vi "Tektronix Model Check.vi"(8 "error in (no error)":errorcluster, 9 "Command String":string, 10 "Oscilloscope Model Tests (3: RF Model?)":u16(ring)=3 items=["Two-channel?", "Digital Model?", "Four-channel?", "RF Model?"], 11 "VISA resource name":refnum<visa-resource-name>) -> (0 "error out":errorcluster, 3 "VISA resource name out":refnum<visa-resource-name>)   [LabVIEW 2017, in "Tektronix DPO MSO 2000 4000 Series.lvlib"]
doc: "Performs a model check on the instrument to verify it supports the commandset that is being written to it. The VI also writes the input command to the instrument."
uses:
  Tektronix DPO MSO 2000 4000 Series.lvlib
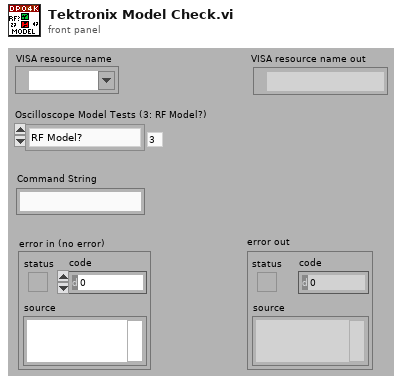
[diagram p1: front panel]
types:
  T1 = typedef "Tektronix DPO MSO 2000 4000 Series.lvlib/Extended User Data.ctl" = cluster{"DPO MSO Series Model":u16}
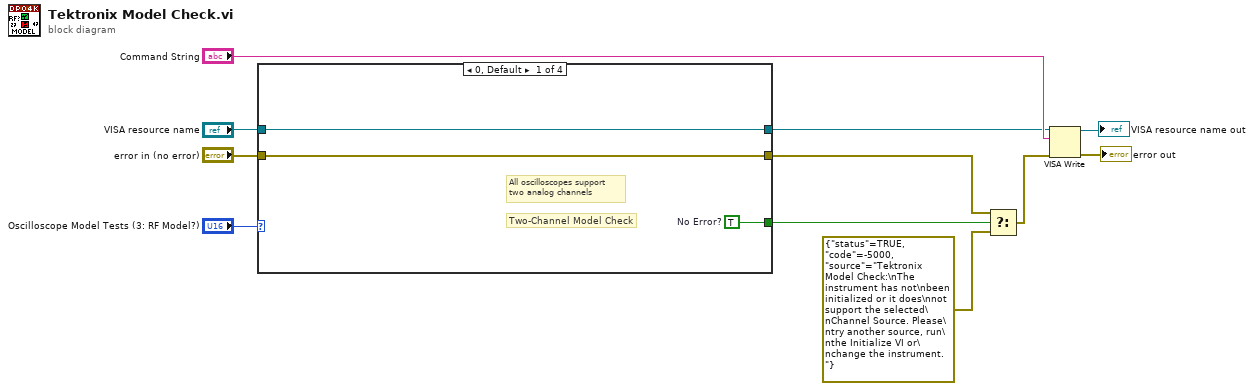
[diagram p0: block diagram]
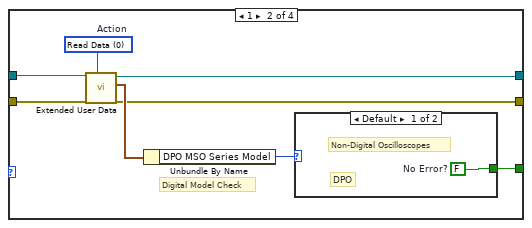
[diagram p2: hidden frame]
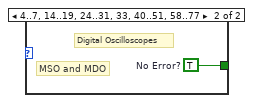
[diagram p3: hidden frame]
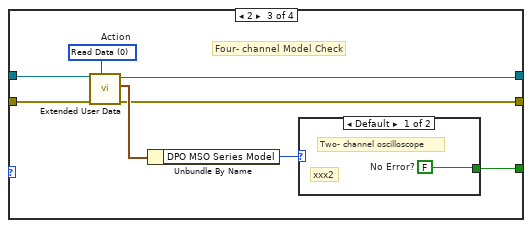
[diagram p4: hidden frame]
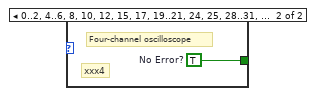
[diagram p5: hidden frame]
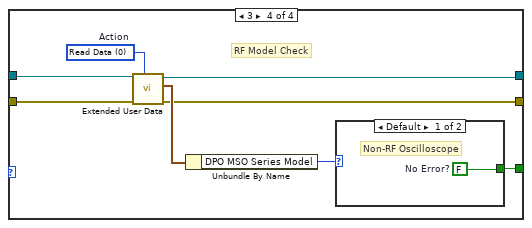
[diagram p6: hidden frame]
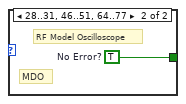
[diagram p7: hidden frame]
diagram:
  n1 = case shown="0, Default" "Oscilloscope Model Tests (3: RF Model?)" {
    tunnel: "VISA resource name" -> [w14 w19 w29 w39]
    tunnel: "error in (no error)" -> [w13 w18 w28 w38]
    tunnel: [w14 w17 w27 w37] -> w7
    tunnel: [w13 w16 w26 w35] -> w6
    tunnel: [w12 w22 w32 w42] -> w5
    frame 0, Default {
      w12 = TRUE  # No Error?
      # "All oscilloscopes support\ntwo analog channels"
      # "Two-Channel Model Check"
    }
    frame 1 {
      w21 = 0 items=["Read Data", "Write Data", "Clear Data", "Clear ALL Data"]  # Action
      # "Digital Model Check"
      n2 = call "Extended User Data.vi"("Action (1: Write Data)"=w21, "error in (no error)"=w18, "VISA resource name"=w19) -> ("error out"=w16:errorcluster, "User Data Out"=w20:T1, "VISA resource name out"=w17:refnum<visa-resource-name>)  [unwired: 6 in]
      n3 = Unbundle By Name(w20) -> ("DPO MSO Series Model"=w15:u16)
      n4 = case shown="Default" w15 {
        tunnel: [w23 w24] -> w22
        frame Default {
          w23 = FALSE  # No Error?
          # "DPO"
          # "Non-Digital Oscilloscopes"
        }
        frame 4..7, 14..19, 24..31, 33, 40..51, 58..77 {
          w24 = TRUE  # No Error?
          # "MSO and MDO"
          # "Digital Oscilloscopes"
        }
      }
    }
    frame 2 {
      w31 = 0 items=["Read Data", "Write Data", "Clear Data", "Clear ALL Data"]  # Action
      # "Four- channel Model Check"
      n5 = call "Extended User Data.vi"("Action (1: Write Data)"=w31, "error in (no error)"=w28, "VISA resource name"=w29) -> ("error out"=w26:errorcluster, "User Data Out"=w30:T1, "VISA resource name out"=w27:refnum<visa-resource-name>)  [unwired: 6 in]
      n6 = Unbundle By Name(w30) -> ("DPO MSO Series Model"=w25:u16)
      n7 = case shown="Default" w25 {
        tunnel: [w33 w34] -> w32
        frame Default {
          w33 = FALSE  # No Error?
          # "xxx2"
          # "Two- channel oscilloscope"
        }
        frame 0..2, 4..6, 8, 10, 12, 15, 17, 19..21, 24, 25, 28..31, 37..42, 46..53, 56..59, 62, 63, 69..77 {
          w34 = TRUE  # No Error?
          # "xxx4"
          # "Four-channel oscilloscope"
        }
      }
    }
    frame 3 {
      w40 = 0 items=["Read Data", "Write Data", "Clear Data", "Clear ALL Data"]  # Action
      # "RF Model Check"
      n8 = call "Extended User Data.vi"("Action (1: Write Data)"=w40, "error in (no error)"=w38, "VISA resource name"=w39) -> ("error out"=w35:errorcluster, "User Data Out"=w41:T1, "VISA resource name out"=w37:refnum<visa-resource-name>)  [unwired: 6 in]
      n9 = Unbundle By Name(w41) -> ("DPO MSO Series Model"=w36:u16)
      n10 = case shown="Default" w36 {
        tunnel: [w43 w44] -> w42
        frame Default {
          w43 = FALSE  # No Error?
          # "Non-RF Oscilloscope"
        }
        frame 28..31, 46..51, 64..77 {
          w44 = TRUE  # No Error?
          # "MDO"
          # "RF Model Oscilloscope"
        }
      }
    }
  }
  n11 = Select(t=w6, s=w5, f=errorcluster {"status"=TRUE, "code"=-5000, "source"="Tektronix Model Check:\nThe instrument has not\nbeen initialized or it does\nnot support the selected\nChannel Source. Please\ntry another source, run\nthe Initialize VI or\nchange the instrument."} ("error out")) -> (s? t:f=w9:errorcluster)
  n12 = VISA Write(VISA resource name=w7, write buffer="Command String", error in (no error)=w9) -> (VISA resource name out=→"VISA resource name out":refnum<visa-resource-name>, error out=→"error out":errorcluster)  [unwired: 1 out]
